vi "Main.vi"(8 "error in (no error)":errorcluster, 11 "Project Refnum":refnum<vi>) -> (0 "error out":errorcluster)   [LabVIEW 2019, in "Project Properties.lvlib"]
doc: "Views VI Properties in the Project Explorer tree for side by side comparison of Project VI settings.\n\nCreated by: Ryan Pacini"
uses:
  Project Properties.lvlib
  State.ctl
  VI Property.ctl
panel:
  in  "Properties Filter":string
  in  "Properties Listbox":i32(listbox)
  in  "Tree":string[](tree)
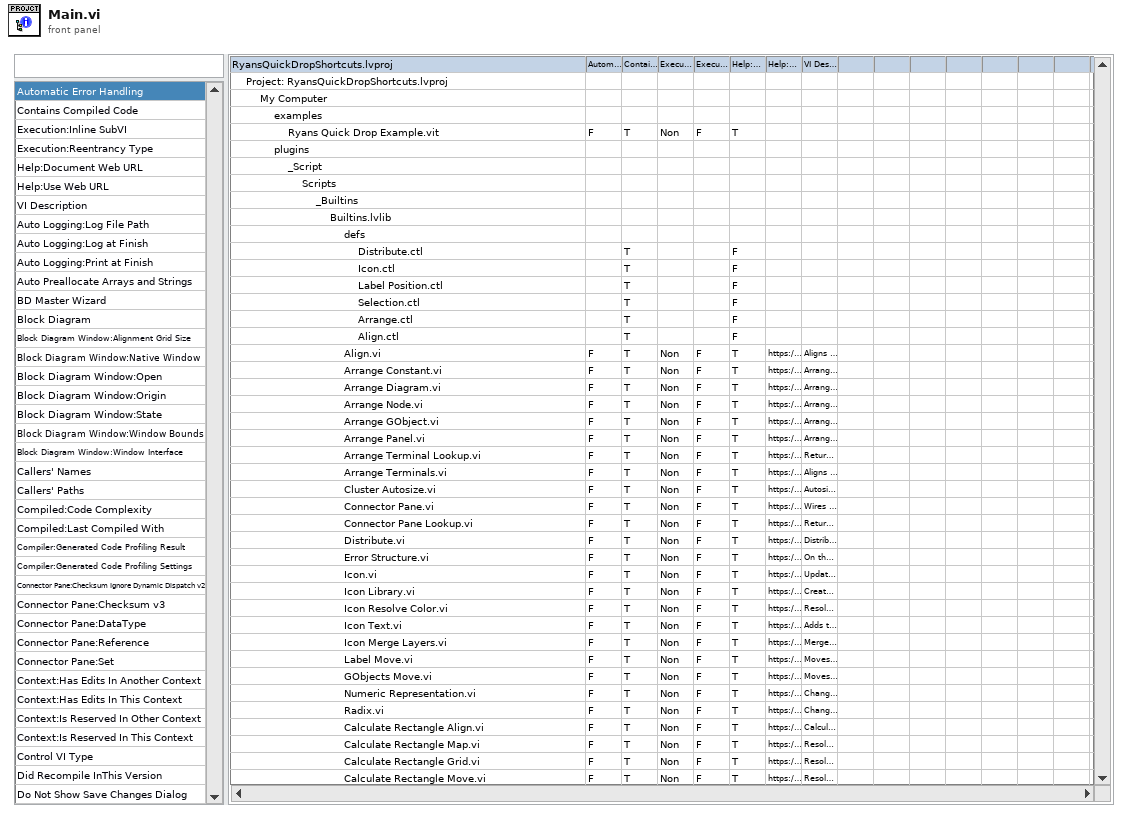
[diagram p1: front panel]
types:
  T1 = typedef "Project Properties.lvlib/State.ctl" = enum8{"property_filter", "property_select", "property_menu_activation", "property_menu_selection", "tree_double_click", "tree_menu_activation", "tree_menu_selection", "export_config"}
  T2 = typedef "Project Properties.lvlib/VI Property.ctl" = enum8{"null", "Auto Logging:Log at Finish", "Auto Logging:Log File Path", "Auto Logging:Print at Finish", "Auto Preallocate Arrays and Strings", "Automatic Error Handling", "BD Master Wizard", "Block Diagram", "Block Diagram Window:Alignment Grid Size", "Block Diagram Window:Native Window", "Block Diagram Window:Open", "Block Diagram Window:Origin", "Block Diagram Window:State", "Block Diagram Window:Window Bounds", "Block Diagram Window:Window Interface", "Callers' Names", "Callers' Paths", "Compiled:Code Complexity", "Compiled:Last Compiled With", "Compiler:Generated Code Profiling Result", "Compiler:Generated Code Profiling Settings", "Connector Pane:Checksum Ignore Dynamic Dispatch v2", "Connector Pane:Checksum v3", "Connector Pane:DataType", "Connector Pane:Reference", "Connector Pane:Set", "Contains Compiled Code", "Context:Has Edits In Another Context", "Context:Has Edits In This Context", "Context:Is Reserved In Other Context", "Context:Is Reserved In This Context", "Control VI Type", "Did Recompile InThis Version", "Do Not Show Save Changes Dialog", "Edit Mode On Open", "Execution highlighting?", "Execution:Allow Debugging", "Execution:Close After Call", "Execution:Compiled With SSE", "Execution:Did Compiler Or User Approve Inlining", "Execution:Inline Enum", "Execution:Inline Is Allowed", "Execution:Inline SubVI", "Execution:Inline SubVI If Possible", "Execution:Is Reentrant", "Execution:Preferred Exec System", "Execution:Priority", "Execution:Reentrancy Type", "Execution:Retain Wire Values", "Execution:Run When Opened", "Execution:Show Front Panel On Call", "Execution:Show Front Panel On Load", "Execution:Shrink Large Buffer Threshold", "Execution:Shrink Large Buffers", "Execution:SSE Runtime Optimization", "Execution:State", "Execution:Suspend On Call", "Expand When Dropped As SubVI", "Front Panel", "Front Panel RefNum TD", "Front Panel Window:Alignment Grid Size", "Front Panel Window:Allow Runtime PopUp", "Front Panel Window:Behavior", "Front Panel Window:Closeable", "Front Panel Window:Custom Title", "Front Panel Window:Highlight Return Button", "Front Panel Window:Is Floating", "Front Panel Window:Is Frontmost", "Front Panel Window:Keep Window Proportions", "Front Panel Window:Minimizable", "Front Panel Window:Minimum Size", "Front Panel Window:Monitor", "Front Panel Window:Native Window", "Front Panel Window:Panel Bounds", "Front Panel Window:Resizable", "Front Panel Window:Run VI Transparently", "Front Panel Window:Show Menu Bar", "Front Panel Window:State", "Front Panel Window:Title", "Front Panel Window:Title Bar Visible", "Front Panel Window:Transparency", "Front Panel Window:Window Bounds", "Front Panel Window:Window Interface", "Has MathScript Nodes", "Help:Document Path", "Help:Document Tag", "Help:Document Web URL", "Help:Examples Exist", "Help:Use Web URL", "Hide Instance VI Caption On Drop", "History:Always Add Comments At Save", "History:Entire Text", "History:Prompt for Comments At Close", "History:Prompt for Comments At Save", "History:Record Application Comments", "History:Revision Number", "History:Use Defaults", "Inline Callees", "Is Clone VI", "Is Generic", "Is In Packed Library", "Is Instance", "Is Probe", "Is Running Interactively", "Is Skinned", "Is System VI", "Is VI Paused?", "Is XNode VI", "Item ID", "Ladder VI Needs Scripting", "Library", "Library:Private", "Library:Version", "Metrics:Advanced", "Metrics:Block Diagram Loaded", "Metrics:Code Size", "Metrics:Front Panel Loaded", "Metrics:Number of clones", "Metrics:Size of Block Diagram", "Metrics:Size of Front Panel", "Metrics:Total Data Size", "Modifications:Block Diagram Mods Bitset", "Modifications:Front Panel Mods Bitset", "Modifications:User Changes", "Modifications:VI Modifications Bitset", "Modifications:VI Signatures", "Modifications:VI User Code GUID", "No Clone If Instance VI", "Number of Non-Proxy Callers", "Overload Info", "Owning Application", "Printing:Block Diagram Scaling?", "Printing:Front Panel Scaling?", "Printing:Header Content:Date Printed?", "Printing:Header Content:Modify Date?", "Printing:Header Content:Page Number?", "Printing:Header Content:VI Icon?", "Printing:Header Content:VI Name?", "Printing:Header Content:VI Path?", "Printing:Margins", "Printing:Page Headers?", "Printing:Page Orientation", "Purgative", "Run-Time Menu Path", "Saved Version", "Statechart:Is Sub Panel Editable", "Statechart:Supress Parse", "Suppress Data Manager", "Suppress Instance VI Halo", "Suppress Transact Info", "Suppress Type Prop", "Tagged And Not Edited", "Terminal Bounds[]", "Tool Bar:Show Abort Button", "Tool Bar:Show Free Run Button", "Tool Bar:Show Run Button", "Tool Bar:Visible", "Tool Kit Attr", "VI Clone Name", "VI Compile Time", "VI Description", "VI Linker Errors", "VI Name", "VI Path", "VI Type"}
  T3 = cluster{"MenuRef":refnum<k9>, "Coords":cluster{"Horizontal":i32, "Vertical":i32}}
  T4 = cluster{"ItemTag":string, "Coords":cluster{"Horizontal":i32, "Vertical":i32}}
  T5 = typedef "Project Properties.lvlib/State Data.ctl" = cluster{"Project Refnum":refnum<vi>, "Tree Refnum":refnum<vi>, "Properties Filter Refnum":refnum<vi>, "Properties Listbox Refnum":refnum<vi>, "Menu Refnum":refnum<k9>, "Project.ini":path, "Properties":T2[], "Render":bool}
  T6 = typedef "LVPoint32TypeDef.ctl" = cluster{"Horizontal":i32, "Vertical":i32}
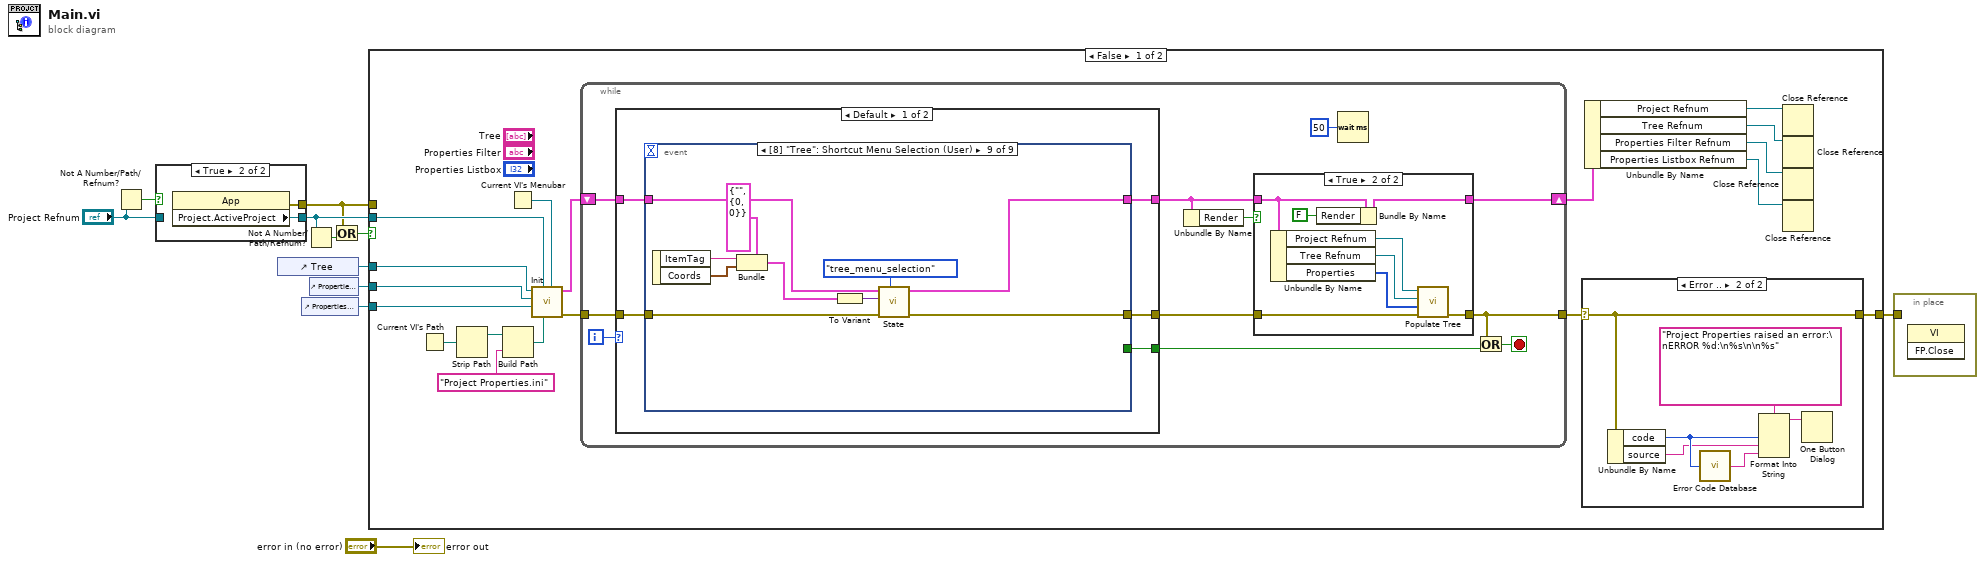
[diagram p0: block diagram]
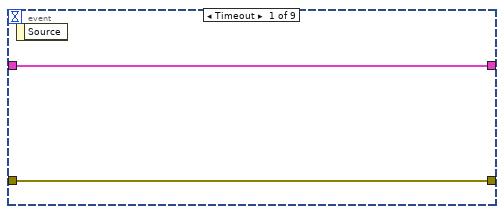
[diagram p3: hidden frame]
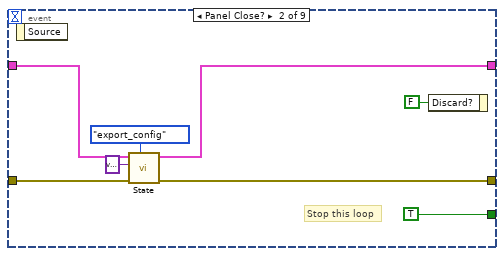
[diagram p4: hidden frame]
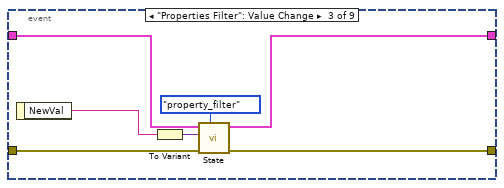
[diagram p5: hidden frame]
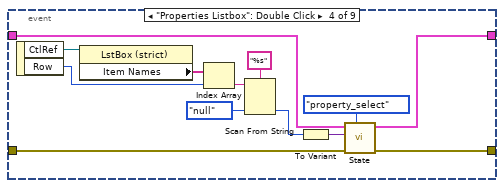
[diagram p6: hidden frame]
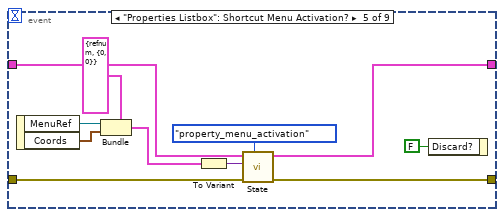
[diagram p7: hidden frame]
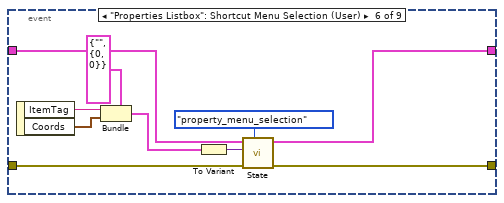
[diagram p8: hidden frame]
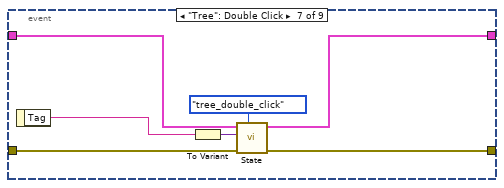
[diagram p9: hidden frame]
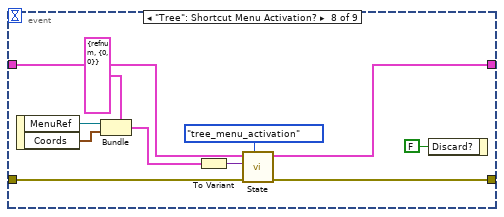
[diagram p10: hidden frame]
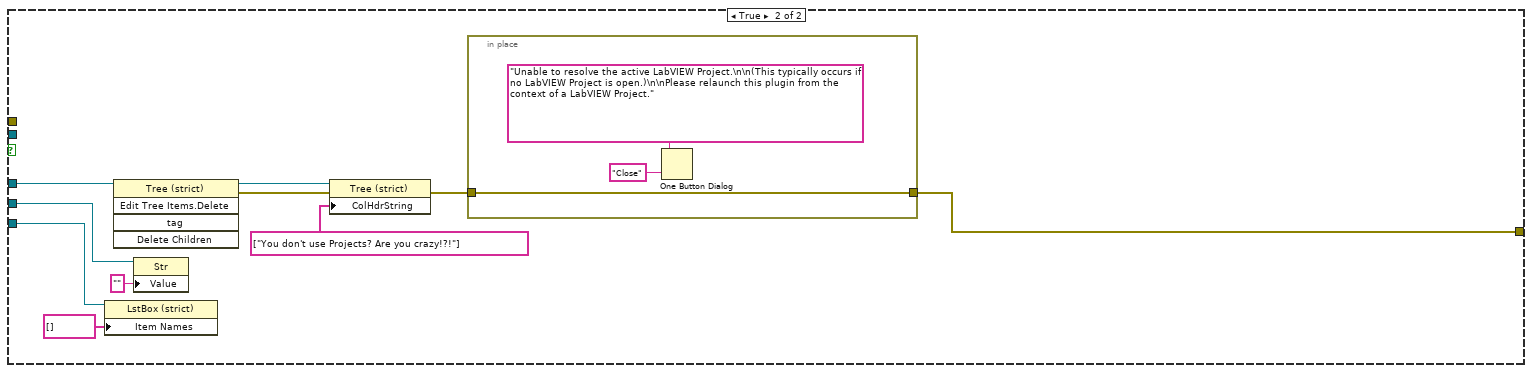
[diagram p13: hidden frame]
diagram:
  n1 = Not A Number/Path/Refnum?(number/path/refnum="Project Refnum") -> (NaN/Path/Refnum?=w9:bool)
  n2 = case shown="True" w9 {
    tunnel: [w12 w14] -> w8
    tunnel: "Project Refnum" -> [w12 _]
    tunnel: [_ w13] -> w6
    frame False {
    }
    frame True {
      n3 = property class="App"() -> (error out=w13:errorcluster, "Project.ActiveProject"=w14:refnum<vi>)  [unwired: 2 in, 1 out]
    }
  }
  n4 = control-ref of="Tree"() -> (w5:refnum<vi>)
  n5 = control-ref of="Properties Listbox"() -> (w3:refnum<vi>)
  n6 = Not A Number/Path/Refnum?(number/path/refnum=w8) -> (NaN/Path/Refnum?=w7:bool)
  n7 = control-ref of="Properties Filter"() -> (w4:refnum<vi>)
  n8 = Or(x=w6, y=w7) -> (x .or. y?=w2:bool)
  n9 = case shown="False" w2 {
    tunnel: w8 -> [w30 _]
    tunnel: w6 -> [_ _]
    tunnel: w5 -> [w19 w156]
    tunnel: w4 -> [w18 w155]
    tunnel: w3 -> [w17 w153]
    tunnel: [w15 w147] -> w1
    frame False {
      n10 = Current VI's Path() -> (path=w23:path)
      n11 = Strip Path(path=w23) -> (stripped path=w24:path)  [unwired: 1 out]
      n12 = Build Path(base path=w24, name or relative path="Project Properties.ini") -> (appended path=w21:path)
      n13 = Current VI's Menubar() -> (w20:refnum<k9>)
      n14 = call "Init.vi"("Menu Refnum"=w20, "Project.ini"=w21, "Project Refnum"=w30, "Properties Listbox Refnum"=w17, "Properties Filter Refnum"=w18, "Tree Refnum"=w19) -> ("error out"=w31:errorcluster, "StateData"=w32:T5)  [unwired: 4 in]
      n15 = while {
        tunnel: w31 -> [w49]
        shift-right: [w46] -> w29
        shift-left: w32 -> [w50]
        tunnel: [w42] -> w16
        i -> [w40]
        stop <- w44 stop-if-true
        n16 = case shown="Default" w40 {
          tunnel: w50 -> [w55 w136]
          tunnel: w49 -> [w54 w135]
          tunnel: [w53 w135] -> w48
          tunnel: [w52 w136] -> w47
          tunnel: [w51 _] -> w43
          frame Default {
            n17 = event shown="[8] \"Tree\": Shortcut Menu Selection (User)" {
              selector: _ -> [_ _ _ _ _ _ _ _ _]
              dyn-events: _ -> [_ _ _ _ _ _ _ _ _]
              timeout: _ -> [_ _ _ _ _ _ _ _ _]
              tunnel: [w57 w59 w70 w84 w95 w105 w109 w123 w133] -> w52
              tunnel: w55 -> [w57 w60 w69 w83 w94 w104 w108 w122 w132]
              tunnel: [w56 w62 w72 w85 w96 w106 w111 w124 w134] -> w53
              tunnel: w54 -> [w56 w61 w71 w74 w91 w101 w110 w119 w129]
              tunnel: [_ TRUE _ _ _ _ _ _ _] -> w51
              event Timeout {
                n18 = event-data() -> ()  [unwired: 1 in, 1 out]
              }
              event Panel Close? {
                # "Stop this loop"
                n19 = event-data() -> ()  [unwired: 1 in, 1 out]
                n20 = call "State.vi"("State"=State."export_config", "error in (no error)"=w61, "Data in"=variant, "StateData in"=w60) -> ("error out"=w62:errorcluster, "StateData out"=w59:T5)  [unwired: 6 in]
                n21 = event-data("Discard?"=FALSE) -> ()  [unwired: 1 in, 1 out]
              }
              event "Properties Filter": Value Change {
                n22 = event-data() -> ("NewVal"=w67:string)  [unwired: 1 in]
                n23 = To Variant(anything=w67) -> (Variant=w66:variant)
                n24 = call "State.vi"("State"=State."property_filter", "error in (no error)"=w71, "Data in"=w66, "StateData in"=w69) -> ("error out"=w72:errorcluster, "StateData out"=w70:T5)  [unwired: 6 in]
              }
              event "Properties Listbox": Double Click {
                n25 = event-data() -> ("CtlRef"=w80:refnum<vi>, "Row"=w77:i32)  [unwired: 1 in]
                n26 = property class="LstBox (strict)"(reference=w80) -> ("Item Names"=w78:string[])  [unwired: 1 in, 2 out]
                n27 = Index Array(array=w78, index=w77) -> (element=w76:string)
                n28 = Scan From String(format string="%s", input string=w76, default 1=VI_Property."null" ("VI Property")) -> (output 1=w73:T2)  [unwired: 2 in, 3 out]
                n29 = To Variant(anything=w73) -> (Variant=w81:variant)
                n30 = call "State.vi"("State"=State."property_select", "error in (no error)"=w74, "Data in"=w81, "StateData in"=w83) -> ("error out"=w85:errorcluster, "StateData out"=w84:T5)  [unwired: 6 in]
              }
              event "Properties Listbox": Shortcut Menu Activation? {
                n31 = event-data() -> ("MenuRef"=w90:refnum<k9>, "Coords"=w89:T6)  [unwired: 1 in]
                n32 = Bundle(cluster=T3 {"MenuRef"=refnum, "Coords"={"Horizontal"=0, "Vertical"=0}}, "MenuRef"=w90, "Coords"=w89) -> (w88:T3)
                n33 = To Variant(anything=w88) -> (Variant=w92:variant)
                n34 = call "State.vi"("State"=State."property_menu_activation", "error in (no error)"=w91, "Data in"=w92, "StateData in"=w94) -> ("error out"=w96:errorcluster, "StateData out"=w95:T5)  [unwired: 6 in]
                n35 = event-data("Discard?"=FALSE) -> ()  [unwired: 1 in, 1 out]
              }
              event "Properties Listbox": Shortcut Menu Selection (User) {
                n36 = event-data() -> ("ItemTag"=w100:string, "Coords"=w99:T6)  [unwired: 1 in]
                n37 = Bundle(cluster=T4 {"ItemTag"="", "Coords"={"Horizontal"=0, "Vertical"=0}}, "ItemTag"=w100, "Coords"=w99) -> (w98:T4)
                n38 = To Variant(anything=w98) -> (Variant=w102:variant)
                n39 = call "State.vi"("State"=State."property_menu_selection", "error in (no error)"=w101, "Data in"=w102, "StateData in"=w104) -> ("error out"=w106:errorcluster, "StateData out"=w105:T5)  [unwired: 6 in]
              }
              event "Tree": Double Click {
                n40 = event-data() -> ("Tag"=w107:string)  [unwired: 1 in]
                n41 = To Variant(anything=w107) -> (Variant=w112:variant)
                n42 = call "State.vi"("State"=State."tree_double_click", "error in (no error)"=w110, "Data in"=w112, "StateData in"=w108) -> ("error out"=w111:errorcluster, "StateData out"=w109:T5)  [unwired: 6 in]
              }
              event "Tree": Shortcut Menu Activation? {
                n43 = event-data() -> ("MenuRef"=w118:refnum<k9>, "Coords"=w117:T6)  [unwired: 1 in]
                n44 = Bundle(cluster=T3 {"MenuRef"=refnum, "Coords"={"Horizontal"=0, "Vertical"=0}}, "MenuRef"=w118, "Coords"=w117) -> (w116:T3)
                n45 = To Variant(anything=w116) -> (Variant=w120:variant)
                n46 = call "State.vi"("State"=State."tree_menu_activation", "error in (no error)"=w119, "Data in"=w120, "StateData in"=w122) -> ("error out"=w124:errorcluster, "StateData out"=w123:T5)  [unwired: 6 in]
                n47 = event-data("Discard?"=FALSE) -> ()  [unwired: 1 in, 1 out]
              }
              event "Tree": Shortcut Menu Selection (User) {
                n48 = event-data() -> ("ItemTag"=w128:string, "Coords"=w127:T6)  [unwired: 1 in]
                n49 = Bundle(cluster=T4 {"ItemTag"="", "Coords"={"Horizontal"=0, "Vertical"=0}}, "ItemTag"=w128, "Coords"=w127) -> (w126:T4)
                n50 = To Variant(anything=w126) -> (Variant=w130:variant)
                n51 = call "State.vi"("State"=State."tree_menu_selection", "error in (no error)"=w129, "Data in"=w130, "StateData in"=w132) -> ("error out"=w134:errorcluster, "StateData out"=w133:T5)  [unwired: 6 in]
              }
            }
          }
          frame 0 {
          }
        }
        n52 = Unbundle By Name(w47) -> ("Render"=w45:bool)
        n53 = case shown="True" w45 {
          tunnel: w48 -> [w138 w146]
          tunnel: w47 -> [w137 w145]
          tunnel: [w137 w141] -> w46
          tunnel: [w138 w139] -> w42
          frame False {
          }
          frame True {
            n54 = Unbundle By Name(w145) -> ("Project Refnum"=w144:refnum<vi>, "Tree Refnum"=w143:refnum<vi>, "Properties"=w142:T2[])
            n55 = Bundle By Name(cluster=w145, "Render"=FALSE) -> (w141:T5)
            n56 = call "Populate Tree.vi"("error in (no error)"=w146, "VI Properties"=w142, "Tree Refnum"=w143, "Project in"=w144) -> ("error out"=w139:errorcluster)  [unwired: 6 in, 1 out]
          }
        }
        n57 = Wait (ms)(milliseconds to wait=u32 50) -> ()  [unwired: 1 out]
        n58 = Or(x=w42, y=w43) -> (x .or. y?=w44:bool)
      }
      n59 = case shown="Error .." w16 {
        selector: w16 -> [w33 w34]
        tunnel: [w33 w34] -> w15
        frame No Error {
        }
        frame Error {
          n60 = Unbundle By Name(w34) -> ("code"=w38:i32, "source"=w36:string)
          n61 = call <vilib>:"Error Code Database.vi"("Error Code"=w38) -> ("Error Text"=w39:string)
          n62 = Format Into String(format string="Project Properties raised an error:\nERROR %d:\n%s\n\n%s", w38, w36, w39) -> (resulting string=w37:string)  [unwired: 2 in, 1 out]
          n63 = One Button Dialog(message=w37) -> ()  [unwired: 1 in, 1 out]
        }
      }
      n64 = Unbundle By Name(w29) -> ("Project Refnum"=w25:refnum<vi>, "Tree Refnum"=w26:refnum<vi>, "Properties Filter Refnum"=w27:refnum<vi>, "Properties Listbox Refnum"=w28:refnum<vi>)
      n65 = Close Reference(reference=w25) -> ()  [unwired: 1 in, 1 out]
      n66 = Close Reference(reference=w26) -> ()  [unwired: 1 in, 1 out]
      n67 = Close Reference(reference=w27) -> ()  [unwired: 1 in, 1 out]
      n68 = Close Reference(reference=w28) -> ()  [unwired: 1 in, 1 out]
    }
    frame True {
      n69 = property class="LstBox (strict)"(reference=w153, "Item Names"=string[] []) -> ()  [unwired: 1 in, 2 out]
      n70 = invoke class="Tree (strict)" method="Edit Tree Items.Delete"(reference=w156) -> (reference out=w151:refnum<vi>, error out=w150:errorcluster)  [unwired: 4 in, 3 out]
      n71 = property class="Str"(reference=w155, "Value"="") -> ()  [unwired: 1 in, 2 out]
      n72 = property class="Tree (strict)"(reference=w151, error in=w150, "ColHdrString"=string[] ["You don't use Projects? Are you crazy!?!"] ("Column Header Strings[]")) -> (error out=w148:errorcluster)  [unwired: 1 out]
      n73 = in-place {
        in-place-border: w148 -> [w157]
        in-place-border: [w157] -> w147
        n74 = One Button Dialog(message="Unable to resolve the active LabVIEW Project.\n\n(This typically occurs if no LabVIEW Project is open.)\n\nPlease relaunch this plugin from the context of a LabVIEW Project." ("source"), button name ("OK")="Close") -> ()  [unwired: 1 out]
      }
    }
  }
  n75 = in-place {
    in-place-border: w1 -> [_]
    n76 = invoke class="VI" method="FP.Close"() -> ()  [unwired: 3 in, 3 out]
  }
  "error out" <- "error in (no error)"
